vi "Nav_Main.vi"(8 "error in":errorcluster, 9 "Robot current position":T2, 10 "Travel Short Distance":bool=TRUE, 11 "Array of path nodes":T1) -> (0 "error out":errorcluster, 3 "Output X and Y":T3)   [LabVIEW 2009, in "Navigation.lvlib"]
uses:
  Navigation.lvlib
  Nav_Cordinates.ctl
  Nav_CordinateArray.ctl
panel:
  out "Y position":dbl
  out "X position":dbl
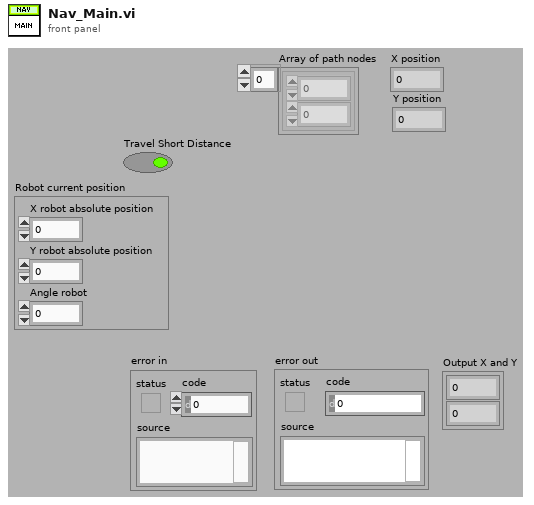
[diagram p1: front panel]
types:
  T1 = typedef "Navigation.lvlib/Nav_CordinateArray.ctl" = cluster{"X position":dbl, "Y position":dbl}[]
  T2 = cluster{"X robot absolute position":dbl, "Y robot absolute position":dbl, "Angle robot":dbl}
  T3 = typedef "Navigation.lvlib/Nav_Cordinates.ctl" = cluster{"X position":dbl, "Y position":dbl}
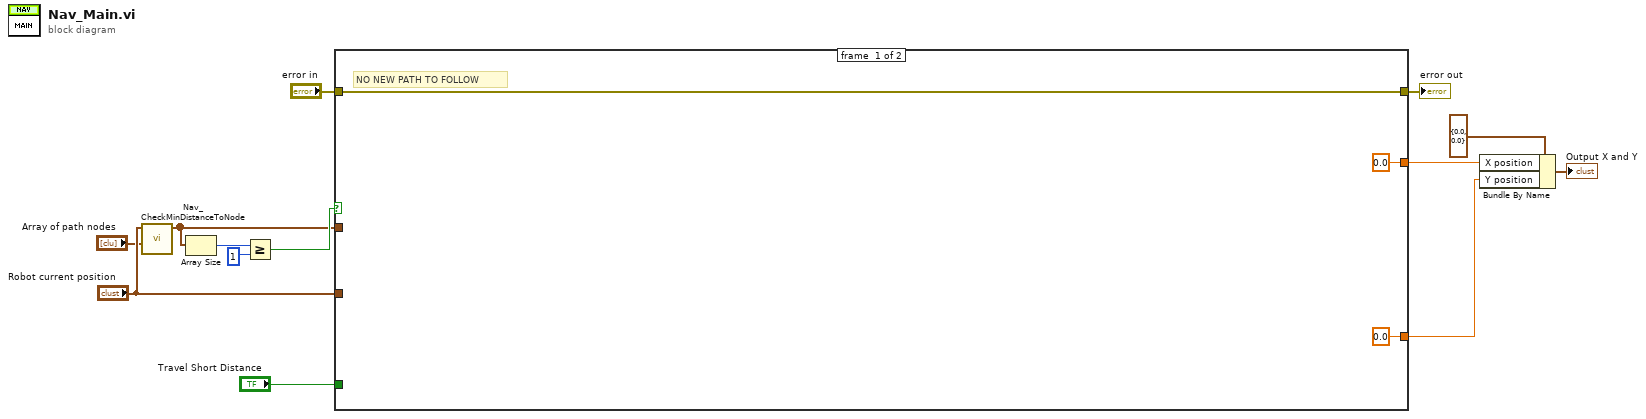
[diagram p0: block diagram]
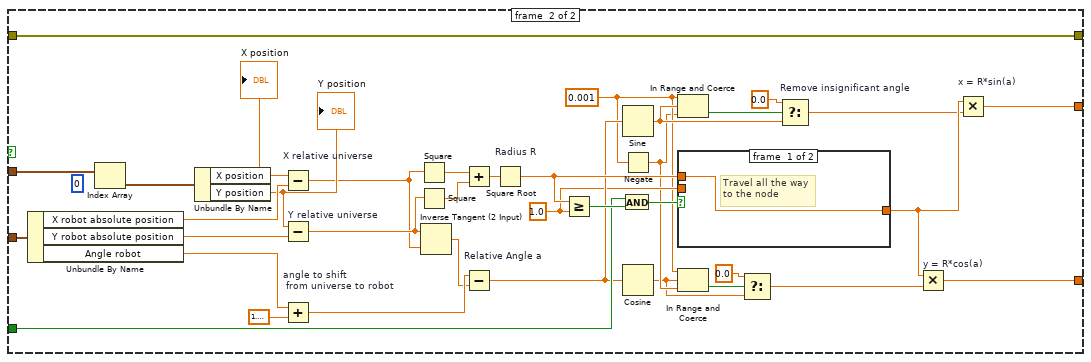
[diagram p2: hidden frame]
diagram:
  n1 = call "Nav_CheckMinDistanceToNode.vi"("Array of path nodes"="Array of path nodes", "Robot current position"="Robot current position") -> ("Coordinates"=w3:T1)  [unwired: 9 in]
  n2 = Array Size(array=w3) -> (size(s)=w7:i32)
  n3 = Greater Or Equal?(x=w7, y=1) -> (x >= y?=w6:bool)
  n4 = case shown="False" w6 {
    tunnel: w3 -> [_ w52]
    tunnel: "error in" -> [w14 w38]
    tunnel: "Robot current position" -> [_ w50]
    tunnel: [0.0 w45] -> w1
    tunnel: [0.0 w44] -> w2
    tunnel: "Travel Short Distance" -> [_ w29]
    tunnel: [w14 w38] -> w11
    frame #0 {
      # "NO NEW PATH TO FOLLOW"
    }
    frame #1 {
      w19 = 0.001 ("y")
      w23 = 1.0 ("y")
      (unwired) 0 ("index")
      n5 = Unbundle By Name(w50) -> ("X robot absolute position"=w48:dbl, "Y robot absolute position"=w46:dbl, "Angle robot"=w42:dbl)
      n6 = Index Array(array=w52) -> (element=w51:cluster{"X position":dbl, "Y position":dbl})  [unwired: 1 in]
      n7 = Unbundle By Name(w51) -> ("X position"=w49:dbl, "Y position"=w47:dbl)
      "X position" <- w49
      "Y position" <- w47
      n8 = Subtract "X relative universe"(x=w49, y=w48) -> (x-y=w33:dbl)
      n9 = Subtract "Y relative universe"(x=w47, y=w46) -> (x-y=w34:dbl)
      n10 = Add "angle to shift\n from universe to robot"(x=w42, y=1.5707963267948966) -> (x+y=w40:dbl)
      n11 = Square(x=w33) -> (x^2=w37:dbl)
      n12 = Square(x=w34) -> (x^2=w35:dbl)
      n13 = Inverse Tangent (2 Input)(1:w33, 2:w34) -> (0:w39:dbl)
      n14 = Add(x=w37, y=w35) -> (x+y=w36:dbl)
      n15 = Subtract "Relative Angle a"(x=w40, y=w39) -> (x-y=w27:dbl)
      n16 = Square Root "Radius R"(x=w36) -> (sqrt(x)=w32:dbl)
      n17 = Greater Or Equal?(x=w32, y=w23) -> (x >= y?=w31:bool)
      n18 = And(x=w29, y=w31) -> (x .and. y?=w30:bool)
      n19 = Sine(x=w27) -> (sin(x)=w21:dbl)
      n20 = Negate(x=w19) -> (-x=w18:dbl)
      n21 = Cosine(x=w27) -> (cos(x)=w17:dbl)
      n22 = In Range and Coerce(upper limit=w19, x=w21, lower limit=w18) -> (In Range?=w22:bool)  [unwired: 1 out]
      n23 = case shown="True" w30 {
        tunnel: w32 -> [w53 _]
        tunnel: [w53 w54] -> w43
        tunnel: w23 -> [_ w54]
        frame #0 {
          # "Travel all the way\nto the node"
        }
        frame #1 {
          # "Set the radius to\none meter and\ntravel that"
        }
      }
      n24 = In Range and Coerce(upper limit=w19, x=w17, lower limit=w18) -> (In Range?=w20:bool)  [unwired: 1 out]
      n25 = Select(t=0.0 ("f"), s=w20, f=w17) -> (s? t:f=w24:dbl)
      n26 = Select "Remove insignificant angle"(t=0.0 ("f"), s=w22, f=w21) -> (s? t:f=w26:dbl)
      n27 = Multiply "y = R*cos(a)"(x=w43, y=w24) -> (x*y=w45:dbl)
      n28 = Multiply "x = R*sin(a)"(x=w43, y=w26) -> (x*y=w44:dbl)
    }
  }
  "error out" <- w11
  n29 = Bundle By Name(cluster=T3 {"X position"=0.0, "Y position"=0.0} ("Navigation.lvlib:Nav_Cordinates"), "X position"=w2, "Y position"=w1) -> (→"Output X and Y":T3)
